vi "CorGetElectd.vi"(8 "error in (no error)":errorcluster, 11 "Cohort in":refnum<class "Cohort.lvclass">) -> (0 "error out":errorcluster, 1 "Pulse Width [ms]":sgl format="%6.2f", 2 "Pulse Frequency [Hz]":sgl format="%6.2f", 4 "Amplitude":sgl[](array[numeric]), 6 "COR Tag":string)   [LabVIEW 2012, in "Cohort.lvclass"]
uses:
  Cohort.lvclass
  Cohort.lvclass/Cohort.ctl
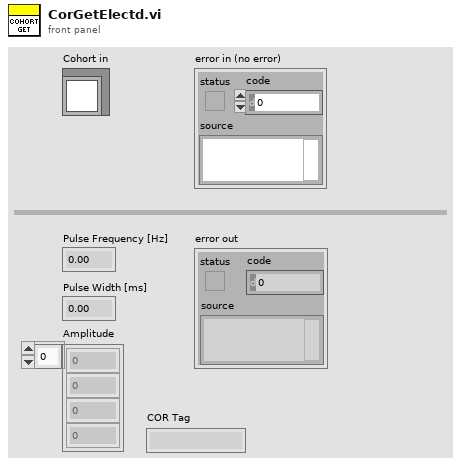
[diagram p1: front panel]
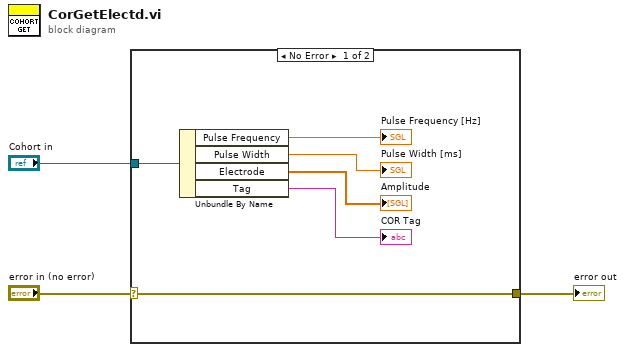
[diagram p0: block diagram]
diagram:
  n1 = case shown="No Error" "error in (no error)" {
    selector: "error in (no error)" -> [w9 w10]
    tunnel: [w9 w10] -> w2
    tunnel: "Cohort in" -> [w8 _]
    frame No Error {
      n2 = Unbundle By Name(w8) -> ("Pulse Frequency"=→"Pulse Frequency [Hz]":sgl, "Pulse Width"=→"Pulse Width [ms]":sgl, "Electrode"=→"Amplitude":sgl[], "Tag"=→"COR Tag":string)
    }
    frame Error {
    }
  }
  "error out" <- w2
